vi "Time.vi"(8 "error in (no error)":errorcluster) -> (0 "error out":errorcluster, 1 "Min":i32, 2 "Hours":i32, 3 "Day":i32, 4 "Time":timestamp, 5 "Str_m":string, 6 "Time":string, 7 "Str_s":string)   [LabVIEW 2017]
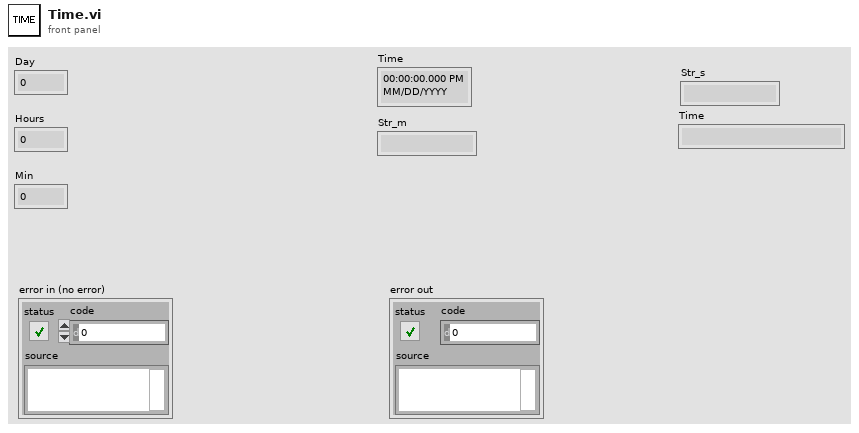
[diagram p1: front panel]
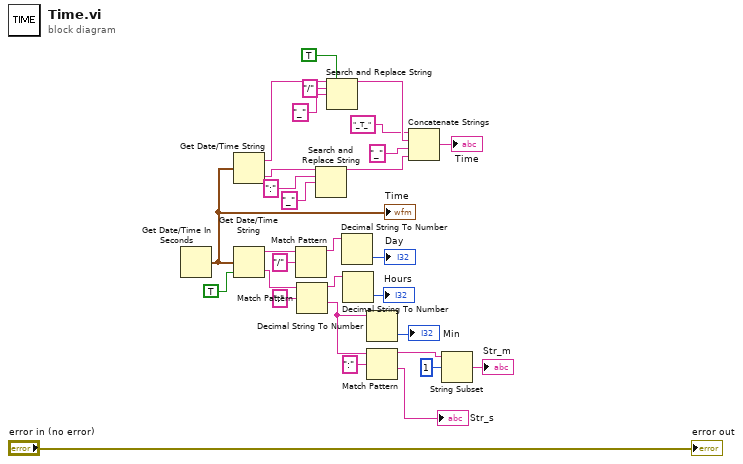
[diagram p0: block diagram]
diagram:
  n1 = Get Date/Time In Seconds() -> (seconds since 1Jan1904=w13:timestamp)
  "Time" <- w13
  n2 = Get Date/Time String(seconds (now)=w13) -> (date string=w4:string, time string=w10:string)  [unwired: 2 in]
  n3 = Get Date/Time String(seconds (now)=w13, want seconds? (F)=TRUE) -> (date string=w28:string, time string=w16:string)  [unwired: 1 in]
  n4 = Match Pattern(string=w28, regular expression="/") -> (before substring=w29:string)  [unwired: 1 in, 3 out]
  n5 = Match Pattern(string=w16, regular expression=":") -> (before substring=w24:string, after substring=w17:string)  [unwired: 1 in, 2 out]
  n6 = Search and Replace String(input string=w10, search string=":", replace string="_" ("replace string (\"\")")) -> (result string=w7:string)  [unwired: 5 in, 3 out]
  n7 = Search and Replace String(replace all?=TRUE ("replace all? (F)"), input string=w4, search string="/", replace string="_" ("replace string (\"\")")) -> (result string=w5:string)  [unwired: 4 in, 3 out]
  n8 = Decimal String To Number(string=w29) -> (number=→"Day":i32)  [unwired: 2 in, 1 out]
  n9 = Decimal String To Number(string=w24) -> (number=→"Hours":i32)  [unwired: 2 in, 1 out]
  n10 = Decimal String To Number(string=w17) -> (number=→"Min":i32)  [unwired: 2 in, 1 out]
  n11 = Match Pattern(string=w17, regular expression=":") -> (before substring=w15:string, after substring=→"Str_s":string)  [unwired: 1 in, 2 out]
  n12 = Concatenate Strings("_T_" ("string"), w5, "_" ("string"), w7) -> (→"Time":string)
  n13 = String Subset(string=w15, offset (0)=1) -> (substring=→"Str_m":string)  [unwired: 1 in]
  "error out" <- "error in (no error)"
